vi "Actor Core.vi"(8 "error in":errorcluster, 11 "Configuration in":refnum<class "Configuration.lvclass">) -> (0 "error out":errorcluster, 3 "Actor out":refnum<class "Actor.lvclass">)   [LabVIEW 2020, in "Configuration.lvlib" / "Configuration.lvclass"]
doc: "(<B>Filename</B>: Actor Framework.lvlib:Actor.lvclass:Actor Core.vi)\n\nReceives messages to the actor, reacts to them, and initiates any error handling that may shut the actor down.\n\nDescendant classes may override this VI to append parallel tasks for the actor to complete while it handles messages. Overrides use the Call Parent Method node."
uses:
  Configuration.lvclass
  C:/Program Files/National Instruments/LabVIEW 2020/vi.lib/ActorFramework/Actor/Actor.lvclass
  <vilib>/ActorFramework/Actor/Actor.lvclass
  Config Actor Core UI Ref.ctl
  <vilib>/ActorFramework/Actor/Actor.lvclass/Actor.ctl
  <vilib>/ActorFramework/Message Enqueuer/Message Enqueuer.lvclass/Message Enqueuer.ctl
  Configuration Messages/Update Config Msg/Update Config Msg.lvclass/Update Config Msg.ctl
  Configuration Messages/Display New Configuration SubPanel Msg/Display New Configuration SubPanel Msg.lvclass/Display New Configuration SubPanel Msg.ctl
  Configuration.lvclass/Configuration.ctl
  <vilib>/ActorFramework/Message Enqueuer/Init from Existing Queue.vi
  <vilib>/ActorFramework/Message Enqueuer/Enqueue.vi
  Configuration Messages/Update Config Msg/Update Config Msg.lvclass
  C:/Program Files/National Instruments/LabVIEW 2020/vi.lib/ActorFramework/Message/Message.lvclass
  Configuration Messages/Save Configuration Msg/Save Configuration Msg.lvclass
  Configuration Messages/Display New Configuration SubPanel Msg/Display New Configuration SubPanel Msg.lvclass
  Configuration Messages/Display Help for Selected Category Msg/Display Help for Highlighted Category Msg.lvclass
  <vilib>/ActorFramework/Stop Msg/Stop Msg.lvclass
  <vilib>/ActorFramework/Message Priority Queue/Priority Enqueue.vi
  <vilib>/ActorFramework/Message Enqueuer/Message Enqueuer.lvclass
panel:
  in  "Categories":i32(listbox)
  out "Title":string
  in  "Help":bool
  in  "OK":bool
  in  "Cancel":bool
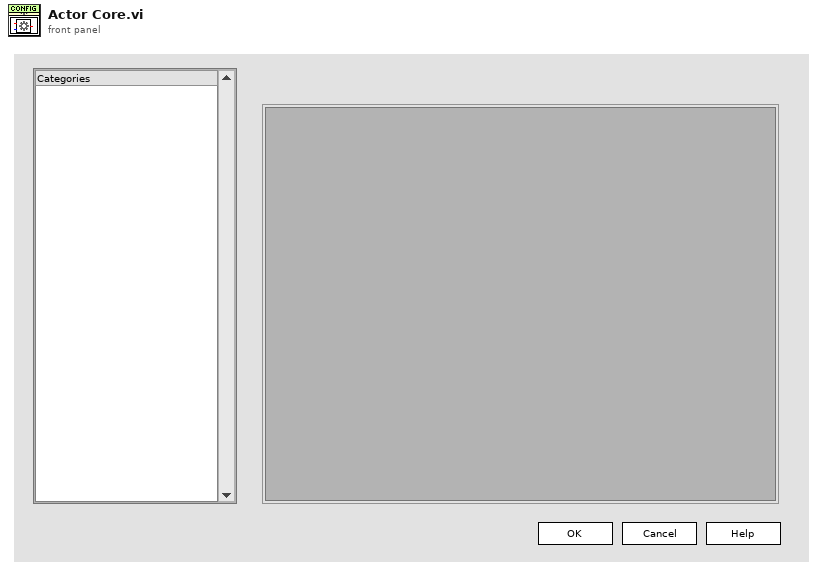
[diagram p1: front panel]
types:
  T1 = typedef "Configuration.lvlib/Configuration.lvclass/Config Actor Core UI Ref.ctl" = cluster{"Title":refnum<vi>, "Sub Panel":refnum<vi>, "OK":refnum<vi>, "Categories":refnum<vi>, "Help":refnum<vi>}
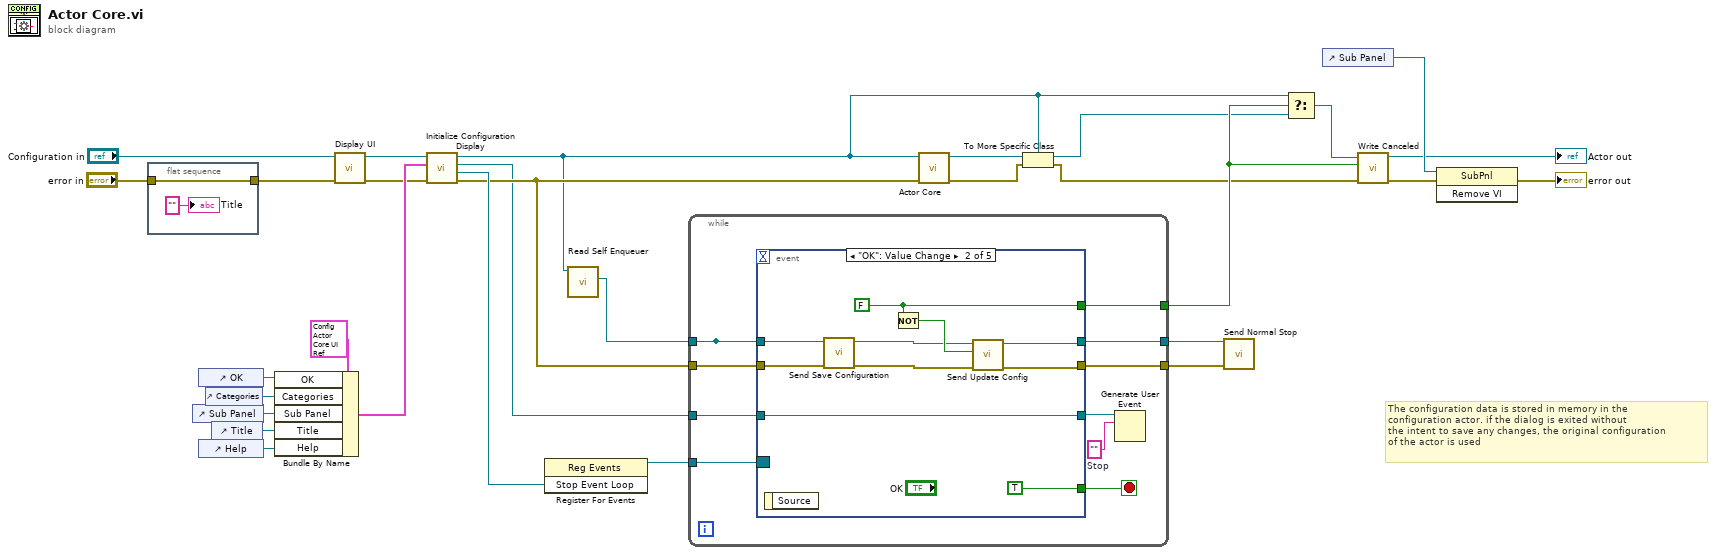
[diagram p0: block diagram]
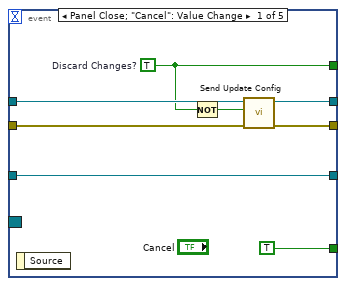
[diagram p2: hidden frame]
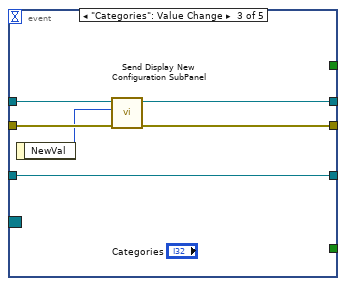
[diagram p3: hidden frame]
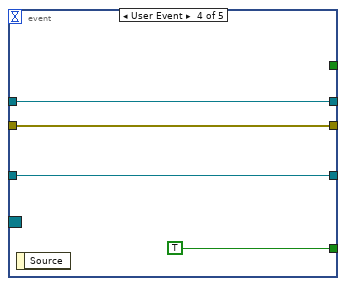
[diagram p4: hidden frame]
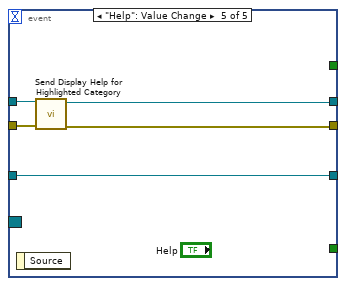
[diagram p5: hidden frame]
diagram:
  # "The configuration data is stored in memory in the\nconfiguration actor. if the dialog is exited without\nthe intent to save any changes, the original configuration\nof the actor is used"
  n1 = flat-sequence {
    tunnel: "error in" -> [w32]
    tunnel: [w32] -> w14
    frame #0 {
      "Title" <- "" ("Title")
    }
  }
  n2 = control-ref of="Sub Panel"() -> (w18:refnum<vi>)
  n3 = control-ref of="OK"() -> (w20:refnum<vi>)
  n4 = control-ref of="Help"() -> (w16:refnum<vi>)
  n5 = control-ref of="Categories"() -> (w19:refnum<vi>)
  n6 = control-ref of="Title"() -> (w17:refnum<vi>)
  n7 = Bundle By Name(cluster=T1 {"Title"=refnum, "Sub Panel"=refnum, "OK"=refnum, "Categories"=refnum, "Help"=refnum} ("Configuration Pane References"), "OK"=w20, "Categories"=w19, "Sub Panel"=w18, "Title"=w17, "Help"=w16) -> (w21:T1)
  n8 = call "Display UI.vi"("error in (no error)"=w14, "Configuration in"="Configuration in") -> ("error out"=w12:errorcluster, "Configuration out"=w13:refnum<class "Configuration.lvclass">)  [unwired: 8 in]
  n9 = call "Initialize Configuration Display.vi"("error in (no error)"=w12, "Configuration Pane References"=w21, "Configuration in"=w13) -> ("error out"=w27:errorcluster, "Stop Event Loop"=w29:refnum<user-event>, "Change Display"=w26:refnum<user-event>, "Configuration out"=w8:refnum<class "Configuration.lvclass">)  [unwired: 5 in]
  n10 = register-events(w29) -> (reference out=w30:refnum<event-registration>)  [unwired: 2 in, 1 out]
  n11 = call <vilib>:"Read Self Enqueuer.vi"("Actor"=w8) -> ("Self Enqueuer"=w28:refnum<class "Message Enqueuer.lvclass">)  [unwired: 10 in]
  n12 = while {
    tunnel: w30 -> [w42]
    tunnel: w28 -> [w35]
    tunnel: w27 -> [w40]
    tunnel: w26 -> [w39]
    tunnel: [w36] -> w11
    tunnel: [w35] -> _
    tunnel: [w34] -> w2
    tunnel: [w33] -> w1
    stop <- w41 stop-if-true
    w37 = ""  # Stop
    n13 = event shown="[1] \"OK\": Value Change" {
      selector: w42 -> [_ _ _ _ _]
      dyn-events: _ -> [_ _ _ _ _]
      timeout: _ -> [_ _ _ _ _]
      tunnel: [TRUE TRUE _ TRUE _] -> w41
      tunnel: w35 -> [w48 w54 w65 w68 w74]
      tunnel: w40 -> [w47 w52 w66 w67 w73]
      tunnel: [w50 w60 w64 w69 w75] -> w38
      tunnel: w39 -> [w50 w60 w64 w69 w75]
      tunnel: [w45 w55 _ _ _] -> w36
      tunnel: [w44 w56 w62 w68 w72] -> w34
      tunnel: [w43 w57 w61 w67 w71] -> w33
      event Panel Close; "Cancel": Value Change {
        w45 = TRUE  # Discard Changes?
        n14 = event-data() -> ()  [unwired: 1 in, 1 out]
        n15 = Not(x=w45) -> (.not. x?=w46:bool)
        n16 = call "Send Update Config.vi"("error in (no error)"=w47, "Update?"=w46, "Message Enqueuer"=w48) -> ("error out"=w43:errorcluster, "Message Enqueuer out"=w44:refnum<class "Message Enqueuer.lvclass">)  [unwired: 7 in]
      }
      event "OK": Value Change {
        w55 = FALSE ("Discard Changes?")
        n17 = event-data() -> ()  [unwired: 1 in, 1 out]
        n18 = call "Send Save Configuration.vi"("error in (no error)"=w52, "Message Enqueuer"=w54) -> ("error out"=w51:errorcluster, "Message Enqueuer out"=w53:refnum<class "Message Enqueuer.lvclass">)  [unwired: 8 in]
        n19 = Not(x=w55) -> (.not. x?=w58:bool)
        n20 = call "Send Update Config.vi"("error in (no error)"=w51, "Update?"=w58, "Message Enqueuer"=w53) -> ("error out"=w57:errorcluster, "Message Enqueuer out"=w56:refnum<class "Message Enqueuer.lvclass">)  [unwired: 7 in]
      }
      event "Categories": Value Change {
        n21 = event-data() -> ("NewVal"=w63:i32)  [unwired: 1 in]
        n22 = call "Send Display New Configuration SubPanel.vi"("error in (no error)"=w66, "ListBox Selection"=w63, "Message Enqueuer"=w65) -> ("error out"=w61:errorcluster, "Message Enqueuer out"=w62:refnum<class "Message Enqueuer.lvclass">)  [unwired: 7 in]
      }
      event User Event {
        n23 = event-data() -> ()  [unwired: 1 in, 1 out]
      }
      event "Help": Value Change {
        n24 = event-data() -> ()  [unwired: 1 in, 1 out]
        n25 = call "Send Display Help for Highlighted Category.vi"("error in (no error)"=w73, "Message Enqueuer"=w74) -> ("error out"=w71:errorcluster, "Message Enqueuer out"=w72:refnum<class "Message Enqueuer.lvclass">)  [unwired: 8 in]
      }
    }
    n26 = Generate User Event(user event=w38, event data cluster=w37) -> ()  [unwired: 2 in, 2 out]
  }
  n27 = call-parent "Actor Core.vi"("error in"=w27, "Actor in"=w8) -> ("error out"=w6:errorcluster, "Actor out"=w9:refnum<class "Actor.lvclass">)  [unwired: 8 in]
  n28 = To More Specific Class(target class=w8, reference=w9, error in=w6) -> (specific class reference=w7:refnum<class "Configuration.lvclass">, error out=w5:errorcluster)
  n29 = call <vilib>:"Send Normal Stop.vi"("error in (no error)"=w1, "Message Enqueuer"=w2) -> ()  [unwired: 9 in, 1 out]
  n30 = Select(t=w8, s=w11, f=w7) -> (s? t:f=w4:refnum<class "Configuration.lvclass">)
  n31 = control-ref of="Sub Panel"() -> (w24:refnum<vi>)
  n32 = call "Write Canceled.vi"("error in (no error)"=w5, "Canceled?"=w11, "Configuration in"=w4) -> ("error out"=w10:errorcluster, "Configuration out"=→"Actor out":refnum<class "Configuration.lvclass">)  [unwired: 7 in]
  n33 = invoke class="SubPnl" method="Remove VI"(reference=w24, error in=w10) -> (error out=→"error out":errorcluster)  [unwired: 1 in, 2 out]
